vi "poly_cast_boolean_notifier_q2n.vi"(2 "boolean queue":refnum<queue>) -> (7 "boolean notifier":T1)   [LabVIEW 2015]
uses:
  cores/boolean_notifier.ctl
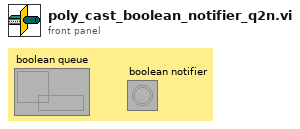
[diagram p1: front panel]
types:
  T1 = typedef "boolean_notifier.ctl" = refnum<k1>
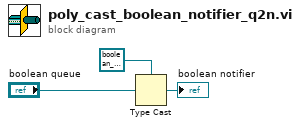
[diagram p0: block diagram]
diagram:
  n1 = Type Cast(type=T1 refnum ("notifier"), x="boolean queue") -> (*(type *) &x=→"boolean notifier":T1)
